vi "_TEST - Send Function Command and Wait on Ret.vi"() -> ()   [LabVIEW 2024, in "EQMF.lvlib" / "Queue Utils.lvlib"]
uses:
  Queue Utils.lvlib
  Q.Element.ctl
panel:
  out "Function Received":string
  in  "AppendStr Cmd":string="AppendStr"
  in  "AppendStr Time Out(ms)":i32=100
  in  "MultNum Funct":string="MultNum"
  in  "AppendStr Delay":i32
  in  "Append Str":string
  in  "AppendStr Funct":bool
  in  "AppendStr Data":string="Test123"
  out "AppendStr Ret":string
  out "Function Error":errorcluster
  in  "Multiplier":dbl=3.0
  in  "MultiNum Time Out(ms)":i32=100
  in  "MultNum Delay":i32
  out "Command Error":errorcluster
  in  "stop":bool
  in  "MultNum Funct":bool
  out "MultNum Ret":dbl
  in  "MultNum Data":dbl=25.0
  # "Function: MultNum"
  # "Function: Append Str"
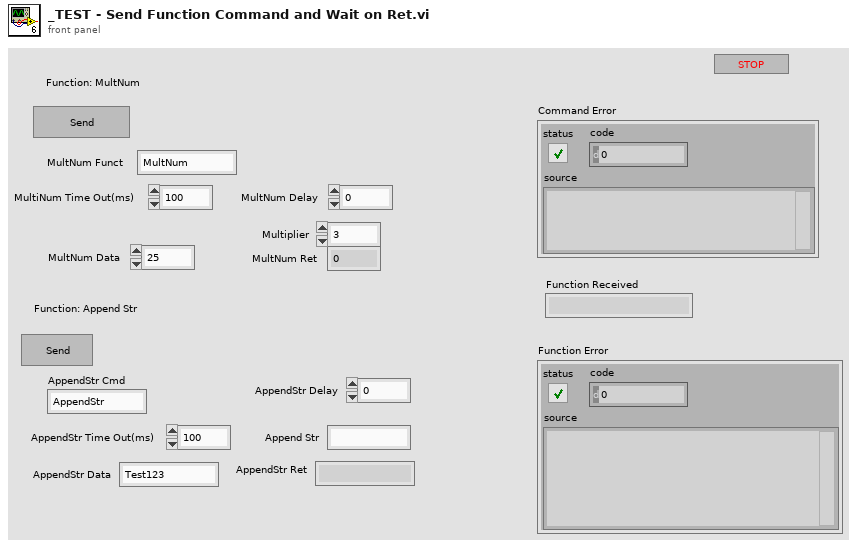
[diagram p1: front panel]
types:
  T1 = typedef "EQMF.lvlib/Queue Utils.lvlib/Q.Element.ctl" = cluster{"Cmd":string, "Sub":string, "Data1":variant, "Data2":variant}
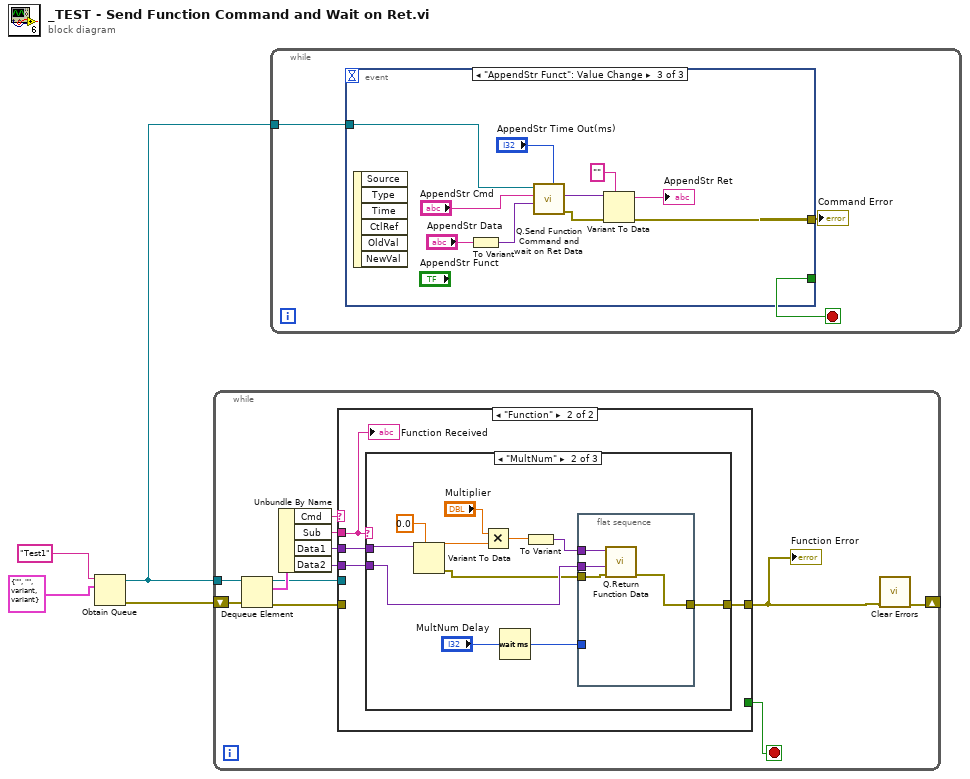
[diagram p0: block diagram]
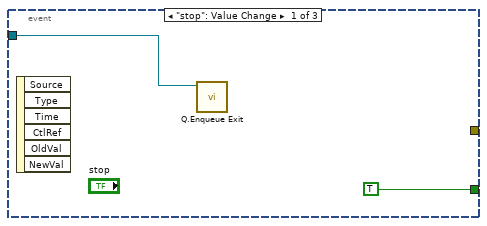
[diagram p2: hidden frame]
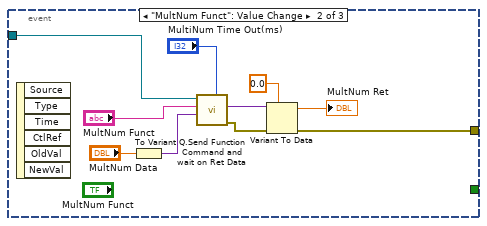
[diagram p3: hidden frame]
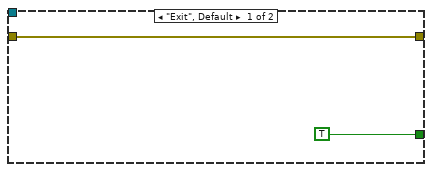
[diagram p4: hidden frame]
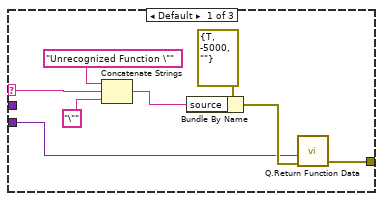
[diagram p5: hidden frame]
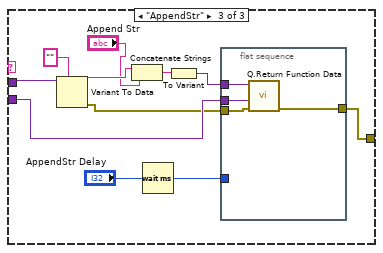
[diagram p6: hidden frame]
diagram:
  n1 = Obtain Queue(name (unnamed)="Test1", element data type=T1 {"Cmd"="", "Sub"="", "Data1"=variant, "Data2"=variant} ("Q.Element")) -> (queue out=w3:refnum<queue>, error out=w4:errorcluster)  [unwired: 3 in, 1 out]
  n2 = while {
    tunnel: w3 -> [w15]
    shift-right: [w6] -> _
    shift-left: w4 -> [w14]
    stop <- w7 stop-if-true
    n3 = Dequeue Element(queue=w15, error in (no error)=w14) -> (queue out=w12:refnum<queue>, element=w16:T1, error out=w13:errorcluster)  [unwired: 1 in, 1 out]
    n4 = Unbundle By Name(w16) -> ("Cmd"=w11:string, "Sub"=w10:string, "Data1"=w9:variant, "Data2"=w8:variant)
    n5 = case shown="\"Function\"" w11 {
      tunnel: w13 -> [w17 _]
      tunnel: w12 -> [_ _]
      tunnel: w10 -> [_ w19]
      tunnel: w9 -> [_ w22]
      tunnel: w8 -> [_ w21]
      tunnel: [TRUE _] -> w7
      tunnel: [w17 w20] -> w5
      frame "Exit", Default {
      }
      frame "Function" {
        n6 = case shown="\"MultNum\"" w19 {
          selector: w19 -> [w26 _ _]
          tunnel: w22 -> [_ w39 w54]
          tunnel: w21 -> [w24 w34 w52]
          tunnel: [w23 w31 w46] -> w20
          frame Default {
            n7 = Concatenate Strings("Unrecognized Function \"", w26, "\"") -> (w29:string)
            n8 = Bundle By Name(cluster=errorcluster {"status"=TRUE, "code"=-5000, "source"=""} ("error constant"), "source"=w29) -> (w25:errorcluster)
            n9 = call "Q.Return Function Data.vi"("error in"=w25, "Data2"=w24) -> ("error out"=w23:errorcluster)  [unwired: 9 in]
          }
          frame "MultNum" {
            n10 = Variant To Data(type=0.0 ("Returned Data"), Variant=w39) -> (data=w37:dbl, error out=w32:errorcluster)  [unwired: 1 in]
            n11 = Multiply(x="Multiplier", y=w37) -> (x*y=w36:dbl)
            n12 = Wait (ms)(milliseconds to wait="MultNum Delay") -> (millisecond timer value=w33:u32)
            n13 = To Variant(anything=w36) -> (Variant=w35:variant)
            n14 = flat-sequence {
              tunnel: w35 -> [w45]
              tunnel: w34 -> [w44]
              tunnel: w33 -> [_]
              tunnel: w32 -> [w43]
              tunnel: [w42] -> w31
              frame #0 {
                n15 = call "Q.Return Function Data.vi"("error in"=w43, "Data2"=w44, "Ret Data"=w45) -> ("error out"=w42:errorcluster)  [unwired: 8 in]
              }
            }
          }
          frame "AppendStr" {
            n16 = Variant To Data(type="" ("Returned Data"), Variant=w54) -> (data=w48:string, error out=w50:errorcluster)  [unwired: 1 in]
            n17 = Concatenate Strings(w48, "Append Str") -> (w49:string)
            n18 = Wait (ms)(milliseconds to wait="AppendStr Delay") -> (millisecond timer value=w51:u32)
            n19 = To Variant(anything=w49) -> (Variant=w53:variant)
            n20 = flat-sequence {
              tunnel: w53 -> [w60]
              tunnel: w52 -> [w59]
              tunnel: w51 -> [_]
              tunnel: w50 -> [w58]
              tunnel: [w57] -> w46
              frame #0 {
                n21 = call "Q.Return Function Data.vi"("error in"=w58, "Data2"=w59, "Ret Data"=w60) -> ("error out"=w57:errorcluster)  [unwired: 8 in]
              }
            }
          }
        }
        "Function Received" <- w19
      }
    }
    "Function Error" <- w5
    n22 = call <vilib>:"Clear Errors.vi"("error in (no error)"=w5) -> ("error out"=w6:errorcluster)  [unwired: 5 in, 1 out]
  }
  n23 = while {
    tunnel: w3 -> [w63]
    stop <- w62 stop-if-true
    n24 = event shown="[2] \"AppendStr Funct\": Value Change" {
      selector: _ -> [_ _ _]
      dyn-events: _ -> [_ _ _]
      timeout: _ -> [_ _ _]
      tunnel: w63 -> [w65 w75 w85]
      tunnel: [TRUE _ _] -> w62
      tunnel: [_ w66 w77] -> w61
      event "stop": Value Change {
        n25 = event-data() -> ()  [unwired: 1 in, 6 out]
        n26 = call "Q.Enqueue Exit.vi"("Q In"=w65) -> ()  [unwired: 9 in, 2 out]
      }
      event "MultNum Funct": Value Change {
        n27 = event-data() -> ()  [unwired: 1 in, 6 out]
        n28 = To Variant(anything="MultNum Data") -> (Variant=w68:variant)
        n29 = call "Q.Send Function Command and wait on Ret Data.vi"("Timeout(ms)"="MultiNum Time Out(ms)", "Data1"=w68, "Cmd"="MultNum Funct", "Q In"=w75) -> ("error out"=w70:errorcluster, "Ret"=w73:variant)  [unwired: 6 in]
        n30 = Variant To Data(error in=w70, type=0.0 ("Returned Data"), Variant=w73) -> (data=→"MultNum Ret":dbl, error out=w66:errorcluster)
      }
      event "AppendStr Funct": Value Change {
        n31 = event-data() -> ()  [unwired: 1 in, 6 out]
        n32 = To Variant(anything="AppendStr Data") -> (Variant=w78:variant)
        n33 = call "Q.Send Function Command and wait on Ret Data.vi"("Timeout(ms)"="AppendStr Time Out(ms)", "Data1"=w78, "Cmd"="AppendStr Cmd", "Q In"=w85) -> ("error out"=w80:errorcluster, "Ret"=w83:variant)  [unwired: 6 in]
        n34 = Variant To Data(error in=w80, type="" ("Returned Data"), Variant=w83) -> (data=→"AppendStr Ret":string, error out=w77:errorcluster)
      }
    }
    "Command Error" <- w61
  }
